vi "GetArduinoResourceName.vi"(8 "error in (no error)":errorcluster) -> (0 "error out":errorcluster, 3 "VISA resource name":refnum<visa-resource-name>)   [LabVIEW 2015]
uses:
  <vilib>/Instr/_visa.llb/VISA Find Search Mode.ctl
  <vilib>/regexp/Match Regular Expression.xnode
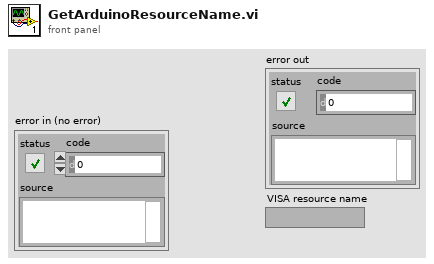
[diagram p1: front panel]
types:
  T1 = typedef "VISA Find Search Mode.ctl" = u32
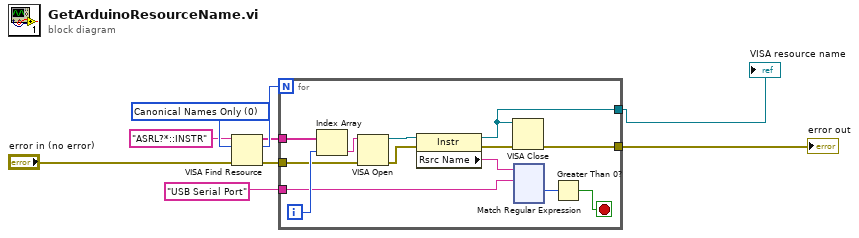
[diagram p0: block diagram]
diagram:
  w8 = T1 0 items=["Canonical Names Only"=0, "Aliases Only"=2, "Include Matching Aliases"=3, "Include All Aliases"=4] ("Search Mode")
  n1 = VISA Find Resource(8:"error in (no error)", 10:w8, 11:"ASRL?*::INSTR" ("expression (\"?*\")")) -> (0:w3:errorcluster, 2:w7:u32, 3:w6:string[])
  n2 = for {
    N: w7 -> [_]
    tunnel: w6 -> [w22]
    tunnel: [w14] -> w2
    tunnel: [w21] -> w1
    tunnel: "USB Serial Port" ("String") -> [w11]
    tunnel: w3 -> [w10]
    i -> [w20]
    stop <- w12 stop-if-true
    n3 = Index Array(array=w22, index=w20) -> (element=w19:string)
    n4 = VISA Open(error in (no error)=w10, VISA resource name=w19) -> (VISA resource name=w18:refnum<visa-resource-name>, error out=w17:errorcluster)  [unwired: 3 in]
    n5 = property class="Instr"(reference=w18, error in=w17) -> (reference out=w14:refnum<visa-resource-name>, error out=w16:errorcluster, "Rsrc Name"=w13:string)
    n6 = VISA Close(VISA resource name=w14, error in (no error)=w16) -> (error out=w21:errorcluster)
    n7 = xnode "Match Regular Expression"("input string"=w13, "regular expression"=w11) -> ("offset past match"=w15:i32)  [unwired: 4 in, 4 out]
    n8 = Greater Than 0?(x=w15) -> (x > 0?=w12:bool)
  }
  "error out" <- w1
  "VISA resource name" <- w2
